vi "Apply Window.vi"(0 "Signal In":fxp<+/-,16,5>, 1 "Window select":T1=enum."None") -> (4 "Windowed Signal Out":fxp<+/-,16,5>)   [LabVIEW 2020]
doc: "This VI applies the specified window function to the input signal, and outputs the modified signal."
uses:
  Type Definitions/Windows.ctl
  <vilib>/Platform/TimedLoop/XDataNode/timing_clust.ctl
  <vilib>/Platform/TimedLoop/XDataNode/nitl_modes.ctl
  <vilib>/Platform/TimedLoop/XDataNode/wakeup.ctl
  <vilib>/rvi/Analysis/common/codeGenErrors/XNode/niFpgaXNodeCodeGenErrorHandle.vi
  <vilib>/rvi/Emulation/niFpgaSctlEmulationGetInTimedLoop.vi
  <vilib>/rvi/Emulation/niFpgaEmulationReportErrorSimple.vi
  <vilib>/rvi/Emulation/niFpgaGetClockAttributes.vi
  <vilib>/rvi/Emulation/niFpgaCriticalErrorInLSC.vi
  <vilib>/rvi/Analysis/measure/window/XNode/niFPGA Scaled Window.xnode
  <vilib>/Platform/TimedLoop/XDataNode/XDataNode.xnode
  <vilib>/rvi/FXPMathLib/basic elements/FxpDiscreteDelay/XNode/nifxpmath_DiscreteDelay.xnode
  <vilib>/rvi/FXPMathLib/FxpMul/XNode/nifxpmath_Multiplier.xnode
  <vilib>/Platform/TimedLoop/XDataNode/XDNodeRunTimeDep.lvlib
  <vilib>/rvi/FXPMathLib/sim/FxpSim.dll
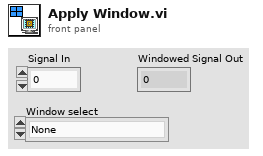
[diagram p1: front panel]
types:
  T1 = typedef "Windows.ctl" = enum16{"Hamming", "Hanning", "None"}
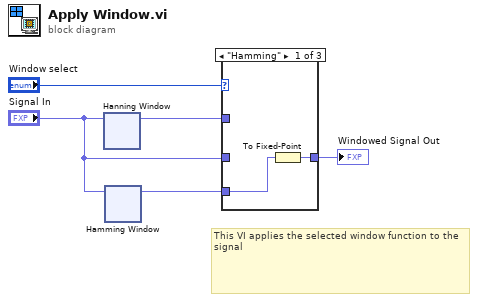
[diagram p0: block diagram]
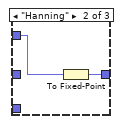
[diagram p2: hidden frame]
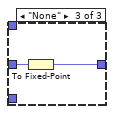
[diagram p3: hidden frame]
diagram:
  # "This VI applies the selected window function to the signal"
  n1 = xnode "Hanning Window"("real data in"="Signal In") -> ("real data out"=w5:fxp<+/-,18,6>)  [unwired: 1 in, 2 out]
  n2 = xnode "Hamming Window"("real data in"="Signal In") -> ("real data out"=w4:fxp<+/-,18,6>)  [unwired: 1 in, 2 out]
  n3 = case shown="\"Hamming\"" "Window select" {
    tunnel: w5 -> [_ w9 _]
    tunnel: [w6 w8 w10] -> w2
    tunnel: w4 -> [w7 _ _]
    tunnel: "Signal In" -> [_ _ w11]
    frame "Hamming" {
      n4 = To Fixed-Point(number=w7) -> (fixed-point=w6:fxp<+/-,16,5>)  [unwired: 1 in]
    }
    frame "Hanning" {
      n5 = To Fixed-Point(number=w9) -> (fixed-point=w8:fxp<+/-,16,5>)  [unwired: 1 in]
    }
    frame "None" {
      n6 = To Fixed-Point(number=w11) -> (fixed-point=w10:fxp<+/-,16,5>)  [unwired: 1 in]
    }
  }
  "Windowed Signal Out" <- w2
